vi "Teleop.vi"(10 "Match Info":T1={"Autonomous Elapsed Seconds"=0.0, "TeleOp Elapsed Seconds"=0.0, "Disabled Elapsed Seconds"=0.0, "Visited Autonomous"=FALSE, "Visited TeleOp"=FALSE, "Visited Disabled"=FALSE, "Autonomous Settings"={"Autonomous Style"=enum."Independent", "VI Refnum"=refnum}}, 11 "Call Context":T2) -> ()   [LabVIEW 2015]
doc: "This VI is called for each TeleOp packet received from the DS where the robot is not disabled. It is often used to read from the joysticks and update I/O or to update setpoints for timed control loops. It should complete and return within 20 milliseconds or it may miss DS packets."
uses:
  <vilib>/Rock Robotics/WPI/DriverStation/WPI_DriverStationDerivedRobotMode.ctl
  <vilib>/Rock Robotics/WPI/DriverStation/WPI_DriverStationMatch Info.ctl
  <vilib>/Rock Robotics/WPI/CAN/TalonSRX/WPI_CANTalonSRX_APIControlMode.ctl
  <vilib>/Rock Robotics/Network Tables/NT Read Boolean.vi
  <vilib>/Rock Robotics/Network Tables/NT Read Number.vi
  <vilib>/Rock Robotics/WPI/Utilities/WPI_GetSetVariantRefNum.vi
  Robot Global Data.vi
panel:
  out "lifter enc":dbl
  out "Auton?":i32
  out "Shooter up to Speed?":bool
  in  "Manually Set Pitch?":bool
  in  "deg":dbl
  out "Valid Target Obtained":bool
  out "Pitch Degrees to Center":dbl
  out "At Angle?":bool
  in  "Manual Mode?":bool
  out "Pitch (Degrees)":dbl
  in  "Move to Target?":bool
  out "Shooter Speed (RPM)":dbl
  out "Pitch":dbl
  out "all currents (A)":dbl[](array[numeric])
  in  "RPM Increments":dbl=0.05 format="%#_13g"
  out "Sample Slider 0":dbl(slide) scale=0.0..5.0
  out "Sample Boolean 1":bool
  out "Sample Boolean 0":bool
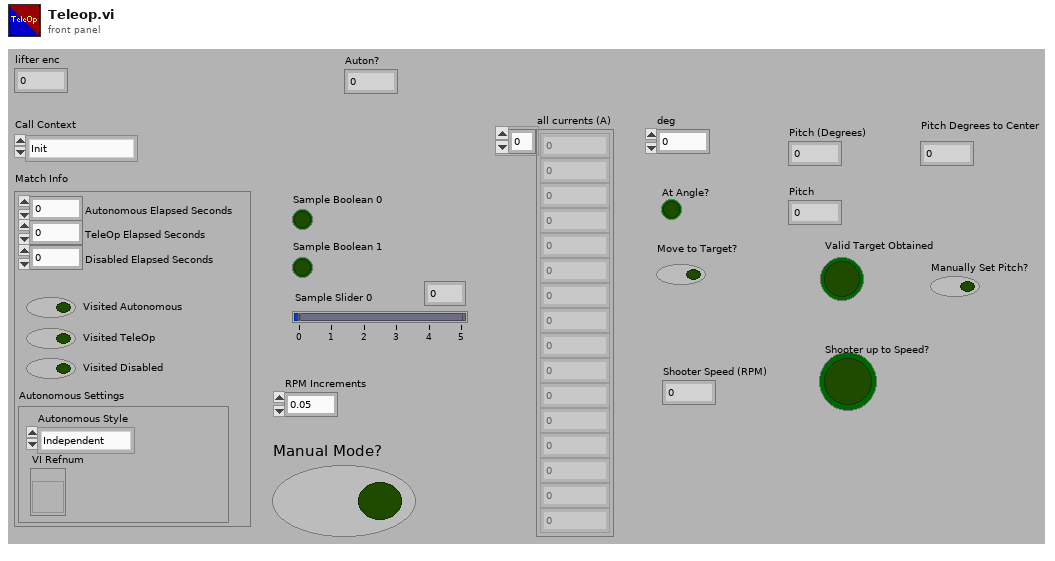
[diagram p1: front panel]
types:
  T1 = typedef "WPI_DriverStationMatch Info.ctl" = cluster{"Autonomous Elapsed Seconds":dbl, "TeleOp Elapsed Seconds":dbl, "Disabled Elapsed Seconds":dbl, "Visited Autonomous":bool, "Visited TeleOp":bool, "Visited Disabled":bool, "Autonomous Settings":cluster{"Autonomous Style":enum16{"Iterative", "Independent"}, "VI Refnum":refnum<vi>}}
  T2 = typedef "WPI_DriverStationDerivedRobotMode.ctl" = enum16{"Init", "Execute", "Stop"}
  T3 = typedef "WPI_GyroDevRef.ctl" = cluster{"DevStatus":errorcluster, "Analog Channel":T4, "Offset":dbl, "Gain (VoltsPerDegree/Second)":dbl, "Gyro Type":enum16{"Analog", "XRS450"}, "Handle":i32, "SPI Bus":T5, "Device Found":bool, "Sample Rate":dbl, "Calibrate On Open":bool}
  T4 = typedef "FPGA_AIChannel.ctl" = enum8{"AI 0", "AI 1", "AI 2", "AI 3", "AI MXP 0", "AI MXP 1", "AI MXP 2", "AI MXP 3", "Invalid"}
  T5 = typedef "spi_bus.ctl" = enum16{"SPI On-Board, CS0", "SPI On-Board, CS1", "SPI On-Board, CS2", "SPI On-Board, CS3", "SPI MXP", "Invalid"}
  T6 = typedef "WPI_DigitalInputDevRef.ctl" = cluster{"DevStatus":errorcluster, "DIO Channel":T7}
  T7 = typedef "FPGA_DIOChannel.ctl" = enum8{"DIO 0", "DIO 1", "DIO 2", "DIO 3", "DIO 4", "DIO 5", "DIO 6", "DIO 7", "DIO 8", "DIO 9", "DIO MXP 0", "DIO MXP 1", "DIO MXP 2", "DIO MXP 3", "DIO MXP 4", "DIO MXP 5", "DIO MXP 6", "DIO MXP 7", "DIO MXP 8", "DIO MXP 9", "DIO MXP 10", "DIO MXP 11", "DIO MXP 12", "DIO MXP 13", "DIO MXP 14", "DIO MXP 15", "Invalid"}
  T8 = typedef "WPI_MotorControlDeviceRef.ctl" = cluster{"DeviceStatus":errorcluster, "Type":T9, "PWM":cluster{"PWM Channel":T10, "DeadBand":T11}, "CAN":cluster{"Device Number":u8, "Control Mode":T12, "Semaphore":T13, "Max Vout":dbl, "TalonSRX Control Mode":T14}, "Invert":bool}
  T9 = typedef "WPI_MotorControlType.ctl" = enum16{"PWM", "CAN", "CANTalonSRX"}
  T10 = typedef "FPGA_DIOPWMChannel.ctl" = enum8{"PWM 0", "PWM 1", "PWM 2", "PWM 3", "PWM 4", "PWM 5", "PWM 6", "PWM 7", "PWM 8", "PWM 9", "PWM MXP 0", "PWM MXP 1", "PWM MXP 2", "PWM MXP 3", "PWM MXP 4", "PWM MXP 5", "PWM MXP 6", "PWM MXP 7", "PWM MXP 8", "PWM MXP 9", "Invalid"}
  T11 = typedef "WPI_PWMDeadband.ctl" = cluster{"Name":string, "maxPositivePwm":i32, "minPositivePwm":i32, "centerPwm":i32, "maxNegativePwm":i32, "minNegativePwm":i32, "angularRange":u16}
  T12 = typedef "WPI_CANJaguar_ControlMode.ctl" = enum8{"Percent VBus", "Current", "Speed", "Position", "Voltage"}
  T13 = typedef "Semaphore RefNum" = refnum<k1>
  T14 = typedef "WPI_CANTalonSRX_APIControlMode.ctl" = enum8{"Percent VBus", "Speed", "Position", "Slave", "Unchanged / Invalid", "Voltage Compensation", "Current", "Motion Profile"}
  T15 = typedef "WPI_JoystickDevRef.ctl" = cluster{"Device":T16}
  T16 = typedef "WPI_JoystickDeviceEnum.ctl" = enum16{"USB 0", "USB 1", "USB 2", "USB 3", "USB 4", "USB 5"}
  T17 = typedef "WPI_ServoDeviceRef.ctl" = cluster{"DeviceStatus":errorcluster, "PWM Channel":T10, "DeadBand":T11}
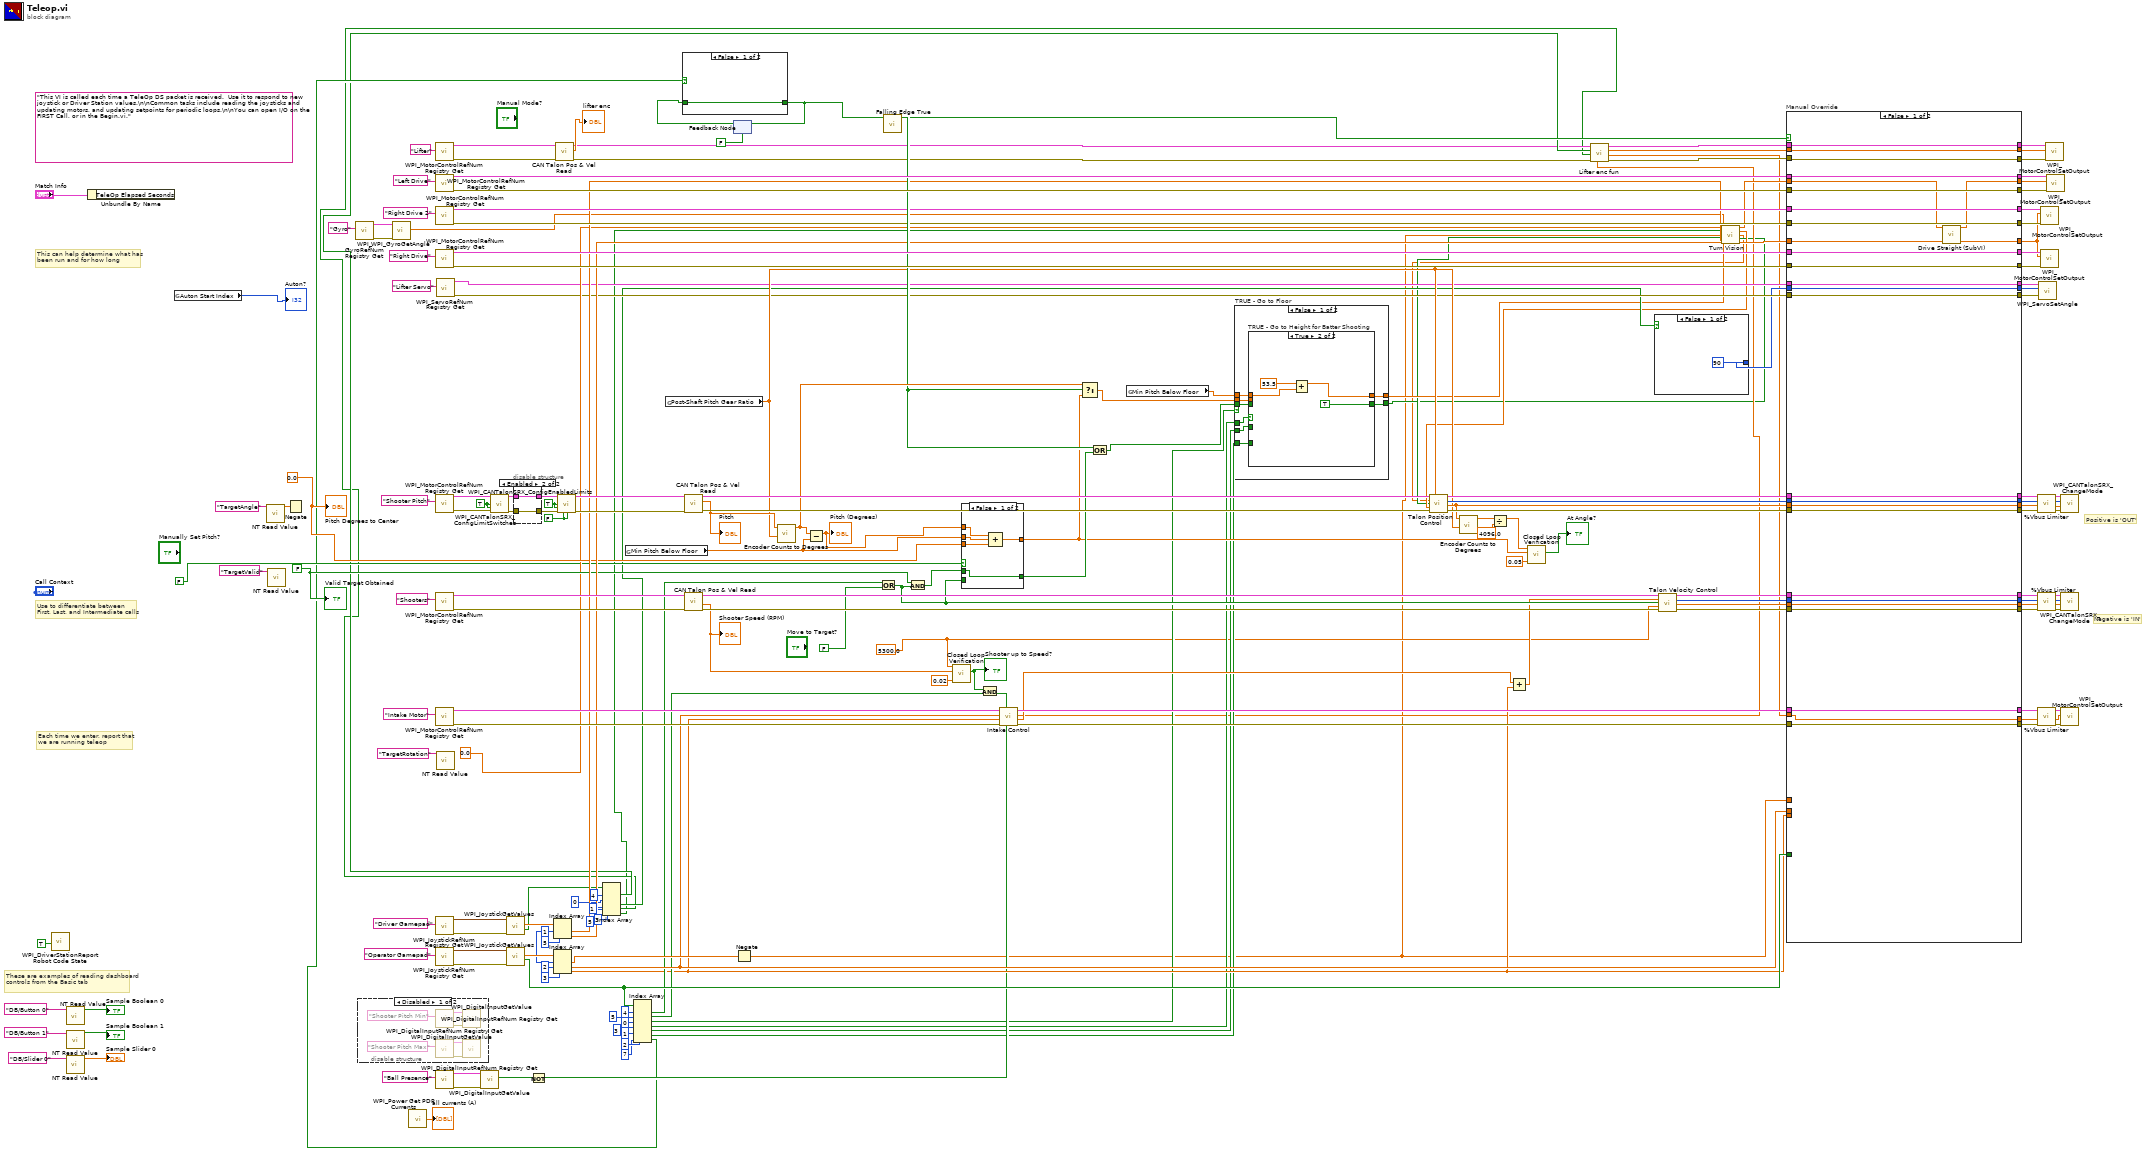
[diagram p0: block diagram]
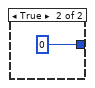
[diagram p2: hidden frame]
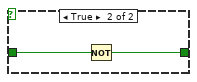
[diagram p3: hidden frame]
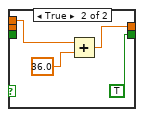
[diagram p5: hidden frame]
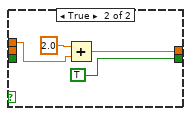
[diagram p6: hidden frame]
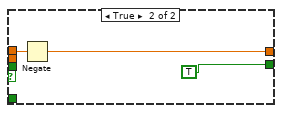
[diagram p7: hidden frame]
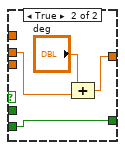
[diagram p8: hidden frame]
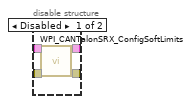
[diagram p9: hidden frame]
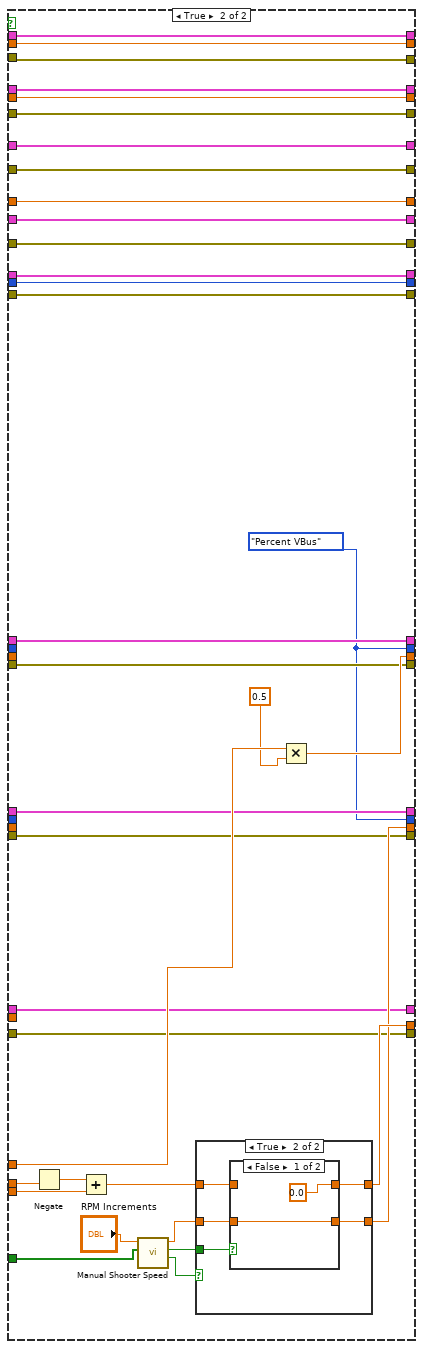
[diagram p11: hidden frame]
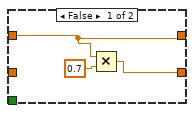
[diagram p12: hidden frame]
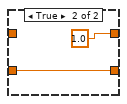
[diagram p13: hidden frame]
diagram:
  w42 = 5300.0 ("Allowable Error Factor")
  w46 = FALSE ("Valid Target Obtained")
  w47 = 0.0 ("Pitch Degrees to Center")
  w144 = FALSE ("Forward Soft Limit Enable")
  w145 = TRUE ("Forward Limit Switch Enable")
  w150 = TRUE ("Forward Limit Switch Normally Open")
  w177 = 1 ("index")
  (unwired) "This VI is called each time a TeleOp DS packet is received.  Use it to respond to new joystick or Driver Station values.\n\nCommon tasks include reading the joysticks and updating motors, and updating setpoints for periodic loops.\n\nYou can open I/O on the FIRST Call, or in the Begin.vi."
  # "Positive is 'OUT'"
  # "Negative is 'IN'"
  # "These are examples of reading dashboard controls from the Basic tab"
  # "Each time we enter, report that\nwe are running teleop"
  # "Use to differentiate between\nFirst, Last, and Intermediate calls"
  # "This can help determine what has\nbeen run and for how long"
  n1 = call <vilib>:"WPI_DriverStationReport Robot Code State.vi"("TeleOp"=TRUE ("Autonomous")) -> ()  [unwired: 10 in, 1 out]
  n2 = call-poly <vilib>:"NT Read Value.vi"("Name"="DB/Button 0" ("refnum name")) -> ("Boolean"=→"Sample Boolean 0":bool)  [unwired: 9 in, 1 out]
  n3 = call-poly <vilib>:"NT Read Value.vi"("Name"="DB/Slider 0" ("refnum name")) -> ("Numeric"=→"Sample Slider 0":dbl)  [unwired: 9 in, 1 out]
  n4 = call-poly <vilib>:"NT Read Value.vi"("Name"="DB/Button 1" ("refnum name")) -> ("Boolean"=→"Sample Boolean 1":bool)  [unwired: 9 in, 1 out]
  n5 = Unbundle By Name("Match Info") -> ()  [unwired: 1 out]
  n6 = global read "Robot Global Data.vi" "Auton Start Index"() -> (→"Auton?":i32)
  n7 = call-poly <vilib>:"NT Read Value.vi"("Name"="TargetAngle") -> ("Numeric"=w86:dbl)  [unwired: 9 in, 1 out]
  n8 = call-poly <vilib>:"NT Read Value.vi"("Name"="TargetValid") -> ()  [unwired: 9 in, 2 out]
  n9 = Negate(x=w86) -> ()  [unwired: 1 out]
  n10 = call <vilib>:"WPI_GyroRefNum Registry Get.vi"("refnum name"="Gyro") -> ("error out"=w67:errorcluster, "GyroDevRef"=w68:T3)  [unwired: 9 in]
  n11 = disable-structure shown="Disabled" {
    frame Disabled {
      n12 = call <vilib>:"WPI_DigitalInputRefNum Registry Get.vi"("refnum name"="Shooter Pitch Min") -> ("error out"=w199:errorcluster, "DigitalInputDevRef"=w200:T6)  [unwired: 9 in]
      n13 = call <vilib>:"WPI_DigitalInputRefNum Registry Get.vi"("refnum name"="Shooter Pitch Max") -> ("error out"=w202:errorcluster, "DigitalInputDevRef"=w201:T6)  [unwired: 9 in]
      n14 = call <vilib>:"WPI_DigitalInputGetValue.vi"("error in (no error)"=w199, "DigitalInputDevRef"=w200) -> ()  [unwired: 7 in, 3 out]
      n15 = call <vilib>:"WPI_DigitalInputGetValue.vi"("error in (no error)"=w202, "DigitalInputDevRef"=w201) -> ()  [unwired: 7 in, 3 out]
    }
    frame Enabled {
    }
  }
  n16 = call <vilib>:"WPI_GyroGetAngle.vi"("error in"=w67, "GyroDevRef"=w68) -> ("Angle"=w66:dbl)  [unwired: 5 in, 4 out]
  n17 = call <vilib>:"WPI_Power Get PDP Currents.vi"() -> ("all currents (A)"=→"all currents (A)":dbl[])  [unwired: 13 in, 2 out]
  n18 = call <vilib>:"WPI_MotorControlRefNum Registry Get.vi"("refnum name"="Lifter") -> ("error out"=w19:errorcluster, "MotorControlDevRef"=w20:T8)  [unwired: 9 in]
  n19 = call <vilib>:"WPI_MotorControlRefNum Registry Get.vi"("refnum name"="Left Drive") -> ("error out"=w165:errorcluster, "MotorControlDevRef"=w170:T8)  [unwired: 9 in]
  n20 = call <vilib>:"WPI_MotorControlRefNum Registry Get.vi"("refnum name"="Right Drive 2") -> ("error out"=w116:errorcluster, "MotorControlDevRef"=w117:T8)  [unwired: 9 in]
  n21 = call <vilib>:"WPI_MotorControlRefNum Registry Get.vi"("refnum name"="Right Drive") -> ("error out"=w164:errorcluster, "MotorControlDevRef"=w169:T8)  [unwired: 9 in]
  n22 = call <vilib>:"WPI_MotorControlRefNum Registry Get.vi"("refnum name"="Shooter Pitch") -> ("error out"=w156:errorcluster, "MotorControlDevRef"=w157:T8)  [unwired: 9 in]
  n23 = call <vilib>:"WPI_MotorControlRefNum Registry Get.vi"("refnum name"="Shooters") -> ("error out"=w151:errorcluster, "MotorControlDevRef"=w168:T8)  [unwired: 9 in]
  n24 = call <vilib>:"WPI_MotorControlRefNum Registry Get.vi"("refnum name"="Intake Motor") -> ("error out"=w92:errorcluster, "MotorControlDevRef"=w93:T8)  [unwired: 9 in]
  n25 = call <vilib>:"WPI_JoystickRefNum Registry Get.vi"("refnum name"="Driver Gamepad") -> ("error out"=w153:errorcluster, "JoystickDevRef"=w197:T15)  [unwired: 1 in, 8 out]
  n26 = call <vilib>:"WPI_JoystickRefNum Registry Get.vi"("refnum name"="Operator Gamepad") -> ("error out"=w154:errorcluster, "JoystickDevRef"=w187:T15)  [unwired: 1 in, 8 out]
  n27 = call <vilib>:"WPI_DigitalInputRefNum Registry Get.vi"("refnum name"="Ball Presence") -> ("error out"=w172:errorcluster, "DigitalInputDevRef"=w171:T6)  [unwired: 9 in]
  n28 = call <vilib>:"WPI_ServoRefNum Registry Get.vi"("refnum name"="Lifter Servo") -> ("error out"=w32:errorcluster, "ServoDeviceRef"=w34:T17)  [unwired: 9 in]
  n29 = call-poly <vilib>:"NT Read Value.vi"("Name"="TargetRotation") -> ()  [unwired: 9 in, 2 out]
  n30 = call <vilib>:"WPI_DigitalInputGetValue.vi"("error in (no error)"=w172, "DigitalInputDevRef"=w171) -> ("Value"=w87:bool)  [unwired: 7 in, 2 out]
  n31 = call <vilib>:"WPI_CANTalonSRX_ConfigLimitSwitches.vi"("CAN Talon SRX Ref"=w157, "Forward Limit Switch Normally Open"=w150, "Reverse Limit Switch Normally Open"=w150, "error in (no error)"=w156) -> ("CAN Talon SRX Ref"=w149:T8, "error out"=w148:errorcluster)  [unwired: 10 in]
  n32 = call <vilib>:"WPI_JoystickGetValues.vi"("error in (no error)"=w153, "JoystickDevRef"=w197) -> ("Buttons"=w70:bool[], "Axes"=w195:dbl[])  [unwired: 5 in, 3 out]
  n33 = call <vilib>:"WPI_JoystickGetValues.vi"("error in (no error)"=w154, "JoystickDevRef"=w187) -> ("Buttons"=w98:bool[], "Axes"=w178:dbl[])  [unwired: 5 in, 3 out]
  n34 = disable-structure shown="Enabled" {
    disable-tunnel: w149 -> [w208 w210]
    disable-tunnel: w148 -> [w207 w209]
    disable-tunnel: [w206 w210] -> w147
    disable-tunnel: [w205 w209] -> w146
    frame Disabled {
      n35 = call <vilib>:"WPI_CANTalonSRX_ConfigSoftLimits.vi"("CAN Talon SRX Ref"=w208, "error in (no error)"=w207) -> ("CAN Talon SRX Ref"=w206:T8, "error out"=w205:errorcluster)  [unwired: 12 in]
    }
    frame Enabled {
    }
  }
  n36 = Not(x=w87) -> (.not. x?=w75:bool)
  n37 = Index Array(array=w195, index #1=w177, index #2=5 ("index")) -> (element #1=w72:dbl, element #2=w74:dbl)
  n38 = Index Array(array=w178, index #1=w177, index #2=2 ("index"), index #3=3 ("index")) -> (element #1=w139:dbl, element #2=w89:dbl, element #3=w78:dbl)
  n39 = call "CAN Talon Pos & Vel Read.vi"("error in (no error)"=w19, "CAN Talon SRX Ref"=w20) -> ("error out"=w14:errorcluster, "Sensor Position"=→"lifter enc":dbl, "CAN Talon SRX Ref"=w16:T8)  [unwired: 5 in, 2 out]
  n40 = call <vilib>:"WPI_CANTalonSRX_ConfigEnabledLimits.vi"("CAN Talon SRX Ref"=w147, "Forward Limit Switch Enable"=w145, "Reverse Limit Switch Enable"=w145, "error in (no error)"=w146, "Forward Soft Limit Enable"=w144, "Reverse Soft Limit Enable"=w144) -> ("CAN Talon SRX Ref"=w155:T8, "error out"=w152:errorcluster)  [unwired: 8 in]
  n41 = Index Array(array=w70, index #1=4 ("index"), index #2=1 ("index"), index #3=0 ("index"), index #4=5 ("index"), index #5=3 ("index")) -> (element #1=w17:bool, element #3=w26:bool, element #4=w12:bool, element #5=w5:bool)  [unwired: 1 out]
  n42 = global read "Robot Global Data.vi" "Min Pitch Below Floor"() -> (w80:dbl)
  n43 = Index Array(array=w98, index #1=4 ("index"), index #2=5 ("index"), index #3=0 ("index"), index #4=3 ("index"), index #5=1 ("index"), index #6=2 ("index"), index #7=7 ("index")) -> (element #1=w83:bool, element #2=w88:bool, element #3=w58:bool, element #4=w56:bool, element #5=w54:bool, element #6=w52:bool, element #7=w39:bool)
  n44 = global read "Robot Global Data.vi" "Post-Shaft Pitch Gear Ratio"() -> (w61:dbl)
  n45 = call "CAN Talon Pos & Vel Read.vi"("error in (no error)"=w152, "CAN Talon SRX Ref"=w155) -> ("error out"=w142:errorcluster, "Sensor Position"=w123:dbl, "CAN Talon SRX Ref"=w143:T8)  [unwired: 5 in, 2 out]
  "Pitch" <- w123
  n46 = call "CAN Talon Pos & Vel Read.vi"("error in (no error)"=w151, "CAN Talon SRX Ref"=w168) -> ("error out"=w106:errorcluster, "Sensor Velocity"=w51:dbl, "CAN Talon SRX Ref"=w107:T8)  [unwired: 5 in, 2 out]
  "Shooter Speed (RPM)" <- w51
  n47 = feedback #1(FALSE) -> (w37:bool)
  n48 = case shown="False" w39 {
    tunnel: w37 -> [w211 w213]
    tunnel: [w211 w212] -> w36
    frame False {
    }
    frame True {
      n49 = Not(x=w213) -> (.not. x?=w212:bool)
    }
  }
  n50 = feedback-in #1(w36) -> ()
  n51 = Negate(x=w139) -> (-x=w2:dbl)
  n52 = call "Encoder Counts to Degrees.vi"("Post-Shaft Gear Ratio"=w61, "Encoder Rotations"=w123) -> ("Degrees"=w122:dbl)  [unwired: 9 in]
  n53 = Subtract(x=w122, y=w80) -> (x-y=w79:dbl)
  "Pitch (Degrees)" <- w79
  n54 = Or(x=w83, y=FALSE) -> (x .or. y?=w82:bool)
  n55 = call "Falling Edge True.vi"("Input"=w36) -> ("Output"=w121:bool)  [unwired: 10 in]
  n56 = And(x=w46, y=w82) -> (x .and. y?=w85:bool)
  n57 = call "Closed Loop Verification.vi"("Allowable Error Factor"=0.02, "Actual"=w51, "Target"=w42) -> ("At Target w/in Allowable Error?"=w48:bool)  [unwired: 8 in]
  "Shooter up to Speed?" <- w48
  n58 = case shown="False" FALSE {
    tunnel: w85 -> [w218 _]
    tunnel: [w218 w222] -> w84
    tunnel: w82 -> [_ w222]
    tunnel: [w214 w220] -> w81
    tunnel: w47 -> [w215 _]
    tunnel: w80 -> [w216 w219]
    tunnel: w79 -> [w217 _]
    frame False {
      n59 = Compound Arithmetic op=ADD(w217, w216, w215) -> (w214:dbl)
    }
    frame True {
      n60 = Compound Arithmetic op=ADD("deg", w219) -> (w220:dbl)
    }
  }
  n61 = And(x=w48, y=w88) -> (x .and. y?=w49:bool)
  n62 = call "Intake Control.vi"("Have Boulder?"=w75, "Shoot?"=w49, "error in (no error)"=w92, "Out %Vbus"=w78, "In %Vbus"=w89, "MotorControlDevRef"=w93) -> ("error out"=w90:errorcluster, "Shooter Modifier"=w76:dbl, "Intake"=w10:dbl, "MotorControlDevRef"=w91:T8)  [unwired: 2 in]
  n63 = Select(t=w122, s=w121, f=w81) -> (s? t:f=w63:dbl)
  n64 = Or(x=w121, y=w84) -> (x .or. y?=w62:bool)
  n65 = global read "Robot Global Data.vi" "Min Pitch Below Floor"() -> (w60:dbl)
  n66 = case "TRUE - Go to Floor" shown="False" w58 {
    tunnel: w63 -> [w229 _]
    tunnel: [w228 w258] -> w8
    tunnel: w62 -> [w227 _]
    tunnel: [w226 TRUE] -> w3
    tunnel: w60 -> [w225 w259]
    tunnel: w56 -> [w230 _]
    tunnel: w54 -> [w224 _]
    tunnel: w52 -> [w223 _]
    frame False {
      n67 = case "TRUE - Go to Height for Batter Shooting" shown="True" w230 {
        tunnel: w229 -> [w234 _]
        tunnel: [w233 w256] -> w228
        tunnel: w227 -> [w236 _]
        tunnel: [w235 TRUE] -> w226
        tunnel: w225 -> [w232 w255]
        tunnel: w224 -> [w237 _]
        tunnel: w223 -> [w231 _]
        frame False {
          n68 = case "TRUE - Go to Height for Defenses" shown="False" w237 {
            tunnel: [w240 TRUE] -> w235
            tunnel: w236 -> [w242 _]
            tunnel: w234 -> [w243 _]
            tunnel: [w239 w251] -> w233
            tunnel: w232 -> [w241 w250]
            tunnel: w231 -> [w238 _]
            frame False {
              n69 = case "TRUE - Height for Shooting\n           from Outer Works" shown="False" w238 {
                tunnel: w243 -> [w244 _]
                tunnel: w242 -> [w245 _]
                tunnel: w241 -> [_ w246]
                tunnel: [w245 TRUE] -> w240
                tunnel: [w244 w247] -> w239
                frame False {
                }
                frame True {
                  n70 = Add(x=w246, y=36.0 ("Degrees")) -> (x+y=w247:dbl)
                }
              }
            }
            frame True {
              n71 = Add(x=2.0 ("Degrees"), y=w250) -> (x+y=w251:dbl)
            }
          }
        }
        frame True {
          n72 = Add(x=53.5 ("Degrees"), y=w255) -> (x+y=w256:dbl)
        }
      }
    }
    frame True {
      n73 = Negate(x=w259) -> (-x=w258:dbl)
    }
  }
  n74 = Add(x=w76, y=w78) -> (x+y=w77:dbl)
  n75 = call "Lifter enc fun.vi"("intake input"=w10, "error in (no error)"=w14, "butten 5"=w12, "butten 4"=w17, "CAN Talon SRX Ref"=w16) -> ("error out"=w13:errorcluster, "Intake output"=w9:dbl, "Lifter output"=w11:dbl, "CAN Talon SRX Ref 2"=w15:T8)  [unwired: 3 in]
  n76 = case shown="False" w26 {
    tunnel: [90 0] -> w29
    frame False {
    }
    frame True {
    }
  }
  n77 = call "Talon Velocity Control.vi"("CAN Talon SRX Ref"=w107, "PercentVoltage"=w77, "Run to Speed?"=w82, "TargetSpeedRPM"=w42, "error in (no error)"=w106) -> ("CAN Talon SRX Ref"=w105:T8, "Control Mode"=w103:T14, "Motor Set"=w102:dbl, "error out"=w104:errorcluster)  [unwired: 7 in]
  n78 = call "Turn Vision.vi"("Angle from camera"=0.0, "AUTO ALIGIN"=w5, "From Current Pitch Positon"=w8, "From Joystick V Align"=w2, "Angle Gyro"=w66, "True from shooter"=w3, "From joystick Right drive"=w74, "From joystick left drive"=w72) -> ("To Left Drive"=w71:dbl, "To Corrected Pitch"=w7:dbl, "To Joystick V Align"=w1:dbl, "True to shooter\n(update position)"=w4:bool, "To Right Drive"=w73:dbl)  [unwired: 3 in]
  n79 = call "Talon Position Control.vi"("CAN Talon SRX Ref"=w143, "Post-Shaft Gear Ratio"=w61, "Joystick"=w1, "Move to Target?"=w4, "Target Degrees"=w7, "error in (no error)"=w142) -> ("CAN Talon SRX Ref"=w141:T8, "Control Mode"=w138:T14, "Encoder Count Target"=w109:dbl, "error out"=w140:errorcluster)  [unwired: 6 in]
  n80 = call "Encoder Counts to Degrees.vi"("Post-Shaft Gear Ratio"=w61, "Encoder Rotations"=w109) -> ("Degrees"=w108:dbl)  [unwired: 9 in]
  n81 = Divide(x=w108, y=4096.0) -> (x/y=w65:dbl)
  n82 = call "Closed Loop Verification.vi"("Allowable Error Factor"=0.05, "Actual"=w81, "Target"=w65) -> ("At Target w/in Allowable Error?"=→"At Angle?":bool)  [unwired: 8 in]
  n83 = case "Manual Override" shown="False" w36 {
    tunnel: w98 -> [_ w324]
    tunnel: w2 -> [_ w323]
    tunnel: [w281 w322] -> w137
    tunnel: w89 -> [_ w319]
    tunnel: w78 -> [_ w318]
    tunnel: [w274 w312] -> w134
    tunnel: [w273 w313] -> w136
    tunnel: w73 -> [w266 w300]
    tunnel: [w263 w302] -> w110
    tunnel: w71 -> [w264 w302]
    tunnel: [w289 w311] -> w112
    tunnel: w170 -> [w289 w311]
    tunnel: w169 -> [w279 w299]
    tunnel: w141 -> [w288 w309]
    tunnel: [w288 w309] -> w163
    tunnel: w105 -> [w287 w308]
    tunnel: [w287 w308] -> w167
    tunnel: w91 -> [w286 w310]
    tunnel: [w286 w310] -> w166
    tunnel: w140 -> [w284 w307]
    tunnel: w104 -> [w283 w306]
    tunnel: w165 -> [w285 w304]
    tunnel: w164 -> [w278 w298]
    tunnel: w90 -> [w282 w305]
    tunnel: [w285 w304] -> w111
    tunnel: [w284 w307] -> w162
    tunnel: [w283 w306] -> w160
    tunnel: [w282 w305] -> w159
    tunnel: w109 -> [w281 _]
    tunnel: w138 -> [w280 _]
    tunnel: [w280 w301] -> w125
    tunnel: [w275 w301] -> w124
    tunnel: [w265 w300] -> w113
    tunnel: [w279 w299] -> w120
    tunnel: [w278 w298] -> w119
    tunnel: [w277 w297] -> w115
    tunnel: w117 -> [w277 w297]
    tunnel: [w276 w296] -> w114
    tunnel: w116 -> [w276 w296]
    tunnel: w103 -> [w275 _]
    tunnel: w102 -> [w274 _]
    tunnel: w9 -> [w273 _]
    tunnel: w34 -> [w272 w295]
    tunnel: [w272 w295] -> w33
    tunnel: w32 -> [w270 w294]
    tunnel: [w270 w294] -> w31
    tunnel: [w271 w293] -> w30
    tunnel: w29 -> [w271 w293]
    tunnel: w15 -> [w269 w292]
    tunnel: [w269 w292] -> w24
    tunnel: [w268 w291] -> w23
    tunnel: w13 -> [w268 w291]
    tunnel: [w267 w290] -> w21
    tunnel: w11 -> [w267 w290]
    frame False {
      n84 = call "Drive Straight (SubVI).vi"("Right Joystick Value"=w266, "Left Joystick Value"=w264) -> ("Right Drive Value"=w265:dbl, "Left Drive Value"=w263:dbl)  [unwired: 8 in]
    }
    frame True {
      w301 = WPI_CANTalonSRX_APIControlMode."Percent VBus" ("Control Mode")
      n85 = Negate(x=w319) -> (-x=w317:dbl)
      n86 = Add(x=w317, y=w318) -> (x+y=w314:dbl)
      n87 = call "Manual Shooter Speed.vi"("Buttons"=w324, "%Vbus Increments"="RPM Increments") -> ("Get to Speed?"=w303:bool, "Shoot?"=w315:bool, "Shooter %Vbus"=w316:dbl)  [unwired: 7 in]
      n88 = case shown="True" w303 {
        tunnel: w316 -> [_ w332]
        tunnel: w315 -> [_ w331]
        tunnel: w314 -> [w326 w330]
        tunnel: [w326 w329] -> w313
        tunnel: [w325 w328] -> w312
        frame False {
          n89 = Multiply(x=w326, y=0.7) -> (x*y=w325:dbl)
        }
        frame True {
          n90 = case shown="False" w331 {
            tunnel: w332 -> [w334 w336]
            tunnel: [w334 w336] -> w328
            tunnel: w330 -> [_ _]
            tunnel: [0.0 1.0] -> w329
            frame False {
            }
            frame True {
            }
          }
        }
      }
      n91 = Multiply(x=w323, y=0.5) -> (x*y=w322:dbl)
    }
  }
  n92 = call "%Vbus Limiter.vi"("error in (no error)"=w162, "Motor Set In"=w137, "Control Mode"=w125, "CAN Talon SRX Ref"=w163) -> ("error out"=w129:errorcluster, "Motor Set Out"=w128:dbl, "Control Mode"=w127:T14, "CAN Talon SRX Ref"=w126:T8)  [unwired: 4 in]
  n93 = call "%Vbus Limiter.vi"("error in (no error)"=w160, "Motor Set In"=w134, "Control Mode"=w124, "CAN Talon SRX Ref"=w167) -> ("error out"=w133:errorcluster, "Motor Set Out"=w132:dbl, "Control Mode"=w131:T14, "CAN Talon SRX Ref"=w130:T8)  [unwired: 4 in]
  n94 = call "%Vbus Limiter.vi"("error in (no error)"=w159, "Motor Set In"=w136, "CAN Talon SRX Ref"=w166) -> ("error out"=w158:errorcluster, "Motor Set Out"=w135:dbl, "CAN Talon SRX Ref"=w161:T8)  [unwired: 5 in, 1 out]
  n95 = call <vilib>:"WPI_ServoSetAngle.vi"("error in (no error)"=w31, "Angle"=w30, "ServoDeviceRef"=w33) -> ()  [unwired: 7 in, 2 out]
  n96 = call <vilib>:"WPI_MotorControlSetOutput.vi"("error in (no error)"=w114, "Output"=w113, "MotorControlDevRef"=w115) -> ()  [unwired: 6 in, 3 out]
  n97 = call <vilib>:"WPI_MotorControlSetOutput.vi"("error in (no error)"=w119, "Output"=w113, "MotorControlDevRef"=w120) -> ()  [unwired: 6 in, 3 out]
  n98 = call <vilib>:"WPI_MotorControlSetOutput.vi"("error in (no error)"=w23, "Output"=w21, "MotorControlDevRef"=w24) -> ()  [unwired: 6 in, 3 out]
  n99 = call <vilib>:"WPI_MotorControlSetOutput.vi"("error in (no error)"=w111, "Output"=w110, "MotorControlDevRef"=w112) -> ()  [unwired: 6 in, 3 out]
  n100 = call <vilib>:"WPI_CANTalonSRX_ChangeMode.vi"("error in (no error)"=w129, "Output"=w128, "Control Mode"=w127, "CAN Talon SRX Ref"=w126) -> ()  [unwired: 6 in, 2 out]
  n101 = call <vilib>:"WPI_CANTalonSRX_ChangeMode.vi"("error in (no error)"=w133, "Output"=w132, "Control Mode"=w131, "CAN Talon SRX Ref"=w130) -> ()  [unwired: 6 in, 2 out]
  n102 = call <vilib>:"WPI_MotorControlSetOutput.vi"("error in (no error)"=w158, "Output"=w135, "MotorControlDevRef"=w161) -> ()  [unwired: 6 in, 3 out]
  "Pitch Degrees to Center" <- w47
  "Valid Target Obtained" <- w46
